vi "low_pass_filter.vi"(9 "gain":dbl, 11 "signal_now":dbl) -> (2 "filtered signal":dbl)   [LabVIEW 2019]
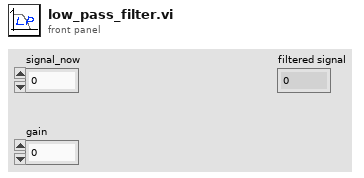
[diagram p1: front panel]
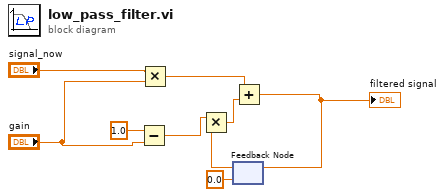
[diagram p0: block diagram]
diagram:
  n1 = Subtract(x=1.0, y="gain") -> (x-y=w3:dbl)
  n2 = Multiply(x="signal_now", y="gain") -> (x*y=w6:dbl)
  n3 = feedback #1(0.0) -> (w2:dbl)
  n4 = Multiply(x=w3, y=w2) -> (x*y=w4:dbl)
  n5 = Add(x=w6, y=w4) -> (x+y=w5:dbl)
  "filtered signal" <- w5
  n6 = feedback-in #1(w5) -> ()
